vi "Set Hue Light Color.vi"() -> ()   [LabVIEW 2013]
doc: "This example demonstrates how to set the RGB color of a Phillips Hue light."
uses:
  vi.lib/MakerHub/Hue/Private/Set Light RGB By ID.vi
  vi.lib/MakerHub/Hue/LMH-Hue.lvlib
panel:
  in  "Color":u32(colorbox)
  in  "Light ID":u8=3
  in  "Stop Button":bool
  in  "Hostname / IP":string
  in  "Username":string
  # "Hue Set Color By ID Example\n\nThis example demonstrates how to set the color of a hue light using the light ID.\n\n1. Enter the Hostname or IP Address of the hue base station.\n2. Enter the Username  you've created on the Hue base station.\n3. Click the Run Arrow.\n4. Enter a Light ID and click the Color box on this LabVIEW front panel to choose \n    the color to set the hue light."
  # "Configure"
  # "Set Color"
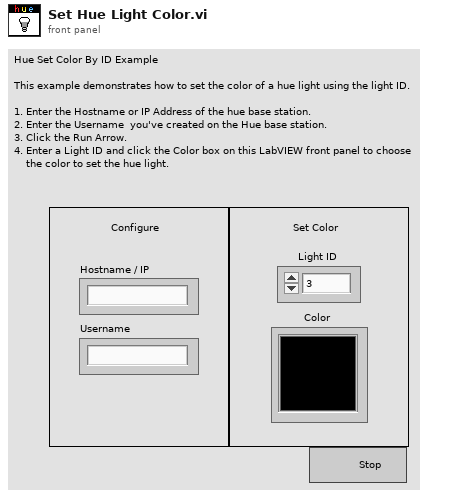
[diagram p1: front panel]
types:
  T1 = typedef "LMH-Hue.lvlib/Hue Ref.ctl" = cluster{"HTTP Session":T2, "Base URL":string, "Lights":T3[]}
  T2 = typedef "LabVIEWHTTPClient.lvlib/ClientHandle.ctl" = refnum<k1>
  T3 = typedef "LMH-Hue.lvlib/Light.ctl" = cluster{"ID":i32, "Name":string}
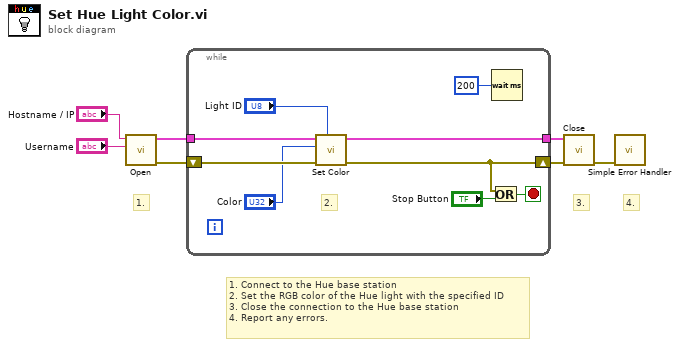
[diagram p0: block diagram]
diagram:
  # "1. Connect to the Hue base station\n2. Set the RGB color of the Hue light with the specified ID\n3. Close the connection to the Hue base station\n4. Report any errors."
  # "4."
  # "3."
  # "1."
  n1 = call "Open.vi"("Username"="Username", "Hostname / IP"="Hostname / IP") -> ("Error Out"=w6:errorcluster, "Hue Config"=w7:T1)  [unwired: 8 in]
  n2 = while {
    tunnel: w7 -> [w15]
    tunnel: [w13] -> w3
    shift-right: [w8] -> w2
    shift-left: w6 -> [w14]
    stop <- w10 stop-if-true
    # "2."
    n3 = call-poly "Set Color.vi"("ID"="Light ID", "Error In"=w14, "Color"="Color", "Hue Config"=w15) -> ("Error Out"=w8:errorcluster, "Hue Config"=w13:T1)  [unwired: 6 in]
    n4 = Or(x=w8, y="Stop Button") -> (x .or. y?=w10:bool)
    n5 = Wait (ms)(milliseconds to wait=u32 200 ("Delay")) -> ()  [unwired: 1 out]
  }
  n6 = call "Close.vi"("Error In"=w2, "Hue Config"=w3) -> ("Error Out"=w1:errorcluster)  [unwired: 9 in]
  n7 = call <vilib>:"Simple Error Handler.vi"("error in (no error)"=w1) -> ()  [unwired: 4 in, 5 out]
